vi "Init Runtime.vi"(8 "error in (no error)":errorcluster, 10 "data allocations":T1, 11 "Parallel Step Config in":refnum<class "Parallel Step Config.lvclass">) -> (0 "error out":errorcluster, 2 "Skip":bool, 3 "Parallel Step Config out":refnum<class "Parallel Step Config.lvclass">)   [LabVIEW 2015, in "Parallel Step Config.lvclass"]
uses:
  Parallel Step Config.lvclass
  <vilib>/NI/Tag Bus Module Framework/channel/data tables.ctl
  <vilib>/NI/Tag Bus/dictionary/data dictionary.lvclass
  <vilib>/NI/Tag Bus/dictionary table pair.ctl
  <vilib>/NI/Tag Bus/table/data table.ctl
  Parallel Step/Parallel Step.lvclass
  Parallel Step Config.lvclass/Parallel Step Config.ctl
  Step/StepState.ctl
  Step/Step State Enum.ctl
  Step/Step Flow Control.ctl
  Step/Step.lvclass
  Step Config/Step Config.lvclass
  <vilib>/NI/Tag Bus/table/data table.lvlib
  <vilib>/NI/Tag Bus/tag bus.lvlib
  <vilib>/NI/Tag Bus Module Framework/channel/TBM channel.lvclass
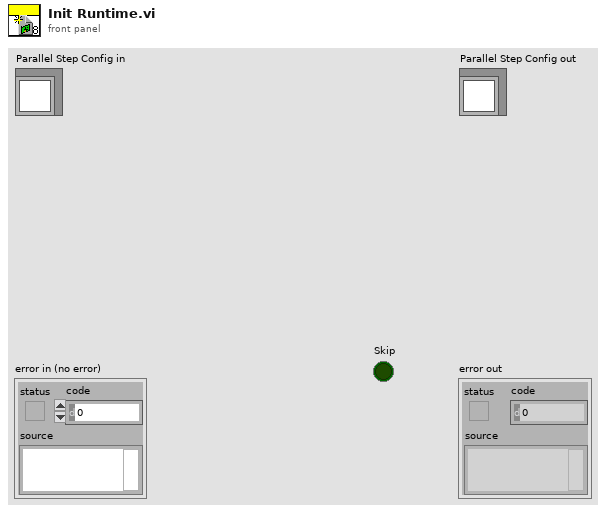
[diagram p1: front panel]
types:
  T1 = typedef "TBM channel.lvclass/data tables.ctl" = cluster{"input data":T2, "processing parameter":T2, "processing result":T2, "output data":T2}
  T2 = typedef "tag bus.lvlib/dictionary table pair.ctl" = cluster{"data dictionary":refnum<class "data dictionary.lvclass">, "data table":T3}
  T3 = typedef "tag bus.lvlib/data table.lvlib/data table.ctl" = cluster{"Double":dbl[], "Single":sgl[], "I64":i64[], "I32":i32[], "I16":i16[], "I8":i8[], "U64":u64[], "U32":u32[], "U16":u16[], "U8":u8[], "Boolean":bool[], "String":string[], "Array of Double":cluster{"DBL Array":dbl[]}[], "Array of Single":cluster{"SGL Array":sgl[]}[], "Array of I64":cluster{"I64 Array":i64[]}[], "Array of I32":cluster{"I32 Array":i32[]}[], "Array of I16":cluster{"I16 Array":i16[]}[], "Array of I8":cluster{"I8 Array":i8[]}[], "Array of U64":cluster{"U64 Array":u64[]}[], "Array of U32":cluster{"U32 Array":u32[]}[], "Array of U16":cluster{"U16 Array":u16[]}[], "Array of U8":cluster{"U8 Array":u8[]}[], "Array of Boolean":cluster{"Boolean Array":bool[]}[], "Array of String":cluster{"String Array":string[]}[]}
  T4 = typedef "Step.lvclass/StepState.ctl" = cluster{"Step State":T5, "Flow Control":T6, "Jump Index":i32}
  T5 = typedef "Step.lvclass/Step State Enum.ctl" = enum16{"Start", "Skipped", "Completed", "Running", "Aborted"}
  T6 = typedef "Step.lvclass/Step Flow Control.ctl" = enum16{"Next Step", "Jump"}
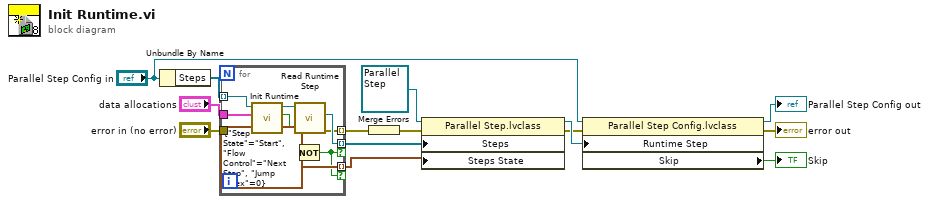
[diagram p0: block diagram]
diagram:
  n1 = Unbundle By Name("Parallel Step Config in") -> ("Steps"=w4:refnum<class "Step Config.lvclass">[])
  n2 = for {
    tunnel: w4 -> [w23] mode=indexing
    tunnel: [w24] -> w11 mode=indexing if=w15
    tunnel: "data allocations" -> [w21]
    tunnel: "error in (no error)" -> [w20]
    tunnel: [w18] -> w10 mode=indexing
    tunnel: [T4 {"Step State"=enum."Start", "Flow Control"=enum."Next Step", "Jump Index"=0} ("Step State")] -> w1 mode=indexing if=w15
    n3 = call-dynamic "Init Runtime.vi"("error in (no error)"=w20, "data allocations"=w21, "Step Config in"=w23) -> ("error out"=w19:errorcluster, "Skip"=w17:bool, "Step Config out"=w22:refnum<class "Step Config.lvclass">)  [unwired: 6 in]
    n4 = Not(x=w17) -> (.not. x?=w15:bool)
    n5 = call-dynamic "Read Runtime Step.vi"("error in (no error)"=w19, "Step Config in"=w22) -> ("error out"=w18:errorcluster, "Step.lvclass"=w24:refnum<class "Step.lvclass">)  [unwired: 7 in, 1 out]
  }
  n6 = Merge Errors(w10) -> (w9:errorcluster)
  n7 = property class="Parallel Step.lvclass"(reference=refnum<class "Parallel Step.lvclass"> refnum ("Parallel Step.lvclass"), error in=w9, "Steps"=w11, "Steps State"=w1) -> (reference out=w12:refnum<class "Parallel Step.lvclass">, error out=w8:errorcluster)
  n8 = property class="Parallel Step Config.lvclass"(reference="Parallel Step Config in", error in=w8, "Runtime Step"=w12) -> (reference out=→"Parallel Step Config out":refnum<class "Parallel Step Config.lvclass">, error out=→"error out":errorcluster, "Skip"=→"Skip":bool)
